vi "GeoData.vi"() -> ()   [LabVIEW 2017] (continued)
MI\tOttawa County\tH1\n49430\t26139\tLamont\tMI\tOttawa County\tH1\n49424\t26139\tHolland\tMI\tOttawa County\tH1\n49415\t26139\tFruitport\tMI\tOttawa County\tH1\n49434\t26139\tMacatawa\tMI\tOttawa County\tH1\n49315\t26139\tByron center\tMI\tOttawa County\tH1\n49330\t26139\tKent city\tMI\tOttawa County\tH1\n49534\t26139\tGrand rapids\tMI\tOttawa County\tH1\n49544\t26139\tGrand rapids\tMI\tOttawa County\tH1\n49422\t26139\tHolland\tMI\tOttawa County\tH1\n49464\t26139\tZeeland\tMI\tOttawa County\tH1\n49448\t26139\tNunica\tMI\tOttawa County\tH1\n49345\t26139\tSparta\tMI\tOttawa County\tH1\n49428\t26139\tJenison\tMI\tOttawa County\tH1\n49401\t26139\tAllendale\tMI\tOttawa County\tH1\n49435\t26139\tMarne\tMI\tOttawa County\tH1\n49404\t26139\tCoopersville\tMI\tOttawa County\tH1\n49417\t26139\tGrand haven\tMI\tOttawa County\tH1\n49460\t26139\tWest olive\tMI\tOttawa County\tH1\n49429\t26139\tJenison\tMI\tOttawa County\tH1\n49403\t26139\tConklin\tMI\tOttawa County\tH1\n49427\t26139\tJamestown\tMI\tOttawa County\tH1\n49318\t26139\tCasnovia\tMI\tOttawa County\tH1\n49451\t26139\tRavenna\tMI\tOttawa County\tH1\n49759\t26141\tMillersburg\tMI\tPresque Isle County\tH1\n49777\t26141\tPresque isle\tMI\tPresque Isle County\tH1\n49743\t26141\tHawks\tMI\tPresque Isle County\tH1\n49707\t26141\tAlpena\tMI\tPresque Isle County\tH1\n49721\t26141\tCheboygan\tMI\tPresque Isle County\tH1\n49746\t26141\tHillman\tMI\tPresque Isle County\tH1\n49776\t26141\tPosen\tMI\tPresque Isle County\tH1\n49779\t26141\tRogers city\tMI\tPresque Isle County\tH1\n49765\t26141\tOnaway\tMI\tPresque Isle County\tH1\n48629\t26143\tHoughton lake\tMI\tRoscommon County\tH1\n48624\t26143\tGladwin\tMI\tRoscommon County\tH1\n48627\t26143\tHiggins lake\tMI\tRoscommon County\tH1\n48653\t26143\tRoscommon\tMI\tRoscommon County\tH1\n48651\t26143\tPrudenville\tMI\tRoscommon County\tH1\n48630\t26143\tHoughton lake heights\tMI\tRoscommon County\tH1\n48656\t26143\tSaint helen\tMI\tRoscommon County\tH1\n48420\t26145\tClio\tMI\tSaginaw County\tH1\n48757\t26145\tReese\tMI\tSaginaw County\tH1\n48417\t26145\tBurt\tMI\tSaginaw County\tH1\n48623\t26145\tFreeland\tMI\tSaginaw County\tH1\n48734\t26145\tFrankenmuth\tMI\tSaginaw County\tH1\n48724\t26145\tCarrollton\tMI\tSaginaw County\tH1\n48457\t26145\tMontrose\tMI\tSaginaw County\tH1\n48601\t26145\tSaginaw\tMI\tSaginaw County\tH1\n48603\t26145\tSaginaw\tMI\tSaginaw County\tH1\n48708\t26145\tBay city\tMI\tSaginaw County\tH1\n48867\t26145\tOwosso\tMI\tSaginaw County\tH1\n48606\t26145\tSaginaw\tMI\tSaginaw County\tH1\n48787\t26145\tFrankenmuth\tMI\tSaginaw County\tH1\n48604\t26145\tSaginaw\tMI\tSaginaw County\tH1\n48608\t26145\tSaginaw\tMI\tSaginaw County\tH1\n48626\t26145\tHemlock\tMI\tSaginaw County\tH1\n48637\t26145\tMerrill\tMI\tSaginaw County\tH1\n48609\t26145\tSaginaw\tMI\tSaginaw County\tH1\n48747\t26145\tMunger\tMI\tSaginaw County\tH1\n48415\t26145\tBirch run\tMI\tSaginaw County\tH1\n48602\t26145\tSaginaw\tMI\tSaginaw County\tH1\n48638\t26145\tSaginaw\tMI\tSaginaw County\tH1\n48722\t26145\tBridgeport\tMI\tSaginaw County\tH1\n48649\t26145\tOakley\tMI\tSaginaw County\tH1\n48460\t26145\tNew lothrop\tMI\tSaginaw County\tH1\n48655\t26145\tSaint charles\tMI\tSaginaw County\tH1\n48607\t26145\tSaginaw\tMI\tSaginaw County\tH1\n48768\t26145\tVassar\tMI\tSaginaw County\tH1\n48841\t26145\tHenderson\tMI\tSaginaw County\tH1\n48616\t26145\tChesaning\tMI\tSaginaw County\tH1\n48807\t26145\tBannister\tMI\tSaginaw County\tH1\n48605\t26145\tSaginaw\tMI\tSaginaw County\tH1\n48614\t26145\tBrant\tMI\tSaginaw County\tH1\n48831\t26145\tElsie\tMI\tSaginaw County\tH1\n48663\t26145\tSaginaw\tMI\tSaginaw County\tH1\n48022\t26147\tEmmett\tMI\tSt. Clair County\tH1\n48014\t26147\tCapac\tMI\tSt. Clair County\tH1\n48041\t26147\tMemphis\tMI\tSt. Clair County\tH1\n48054\t26147\tEast china\tMI\tSt. Clair County\tH1\n48002\t26147\tAllenton\tMI\tSt. Clair County\tH1\n48064\t26147\tCasco\tMI\tSt. Clair County\tH1\n48049\t26147\tNorth street\tMI\tSt. Clair County\tH1\n48060\t26147\tPort huron\tMI\tSt. Clair County\tH1\n48444\t26147\tImlay city\tMI\tSt. Clair County\tH1\n48023\t26147\tFair haven\tMI\tSt. Clair County\tH1\n48032\t26147\tJeddo\tMI\tSt. Clair County\tH1\n48003\t26147\tAlmont\tMI\tSt. Clair County\tH1\n48027\t26147\tGoodells\tMI\tSt. Clair County\tH1\n48061\t26147\tPort huron\tMI\tSt. Clair County\tH1\n48040\t26147\tMarysville\tMI\tSt. Clair County\tH1\n48416\t26147\tBrown city\tMI\tSt. Clair County\tH1\n48006\t26147\tAvoca\tMI\tSt. Clair County\tH1\n48039\t26147\tMarine city\tMI\tSt. Clair County\tH1\n48001\t26147\tAlgonac\tMI\tSt. Clair County\tH1\n48028\t26147\tHarsens island\tMI\tSt. Clair County\tH1\n48004\t26147\tAnchorville\tMI\tSt. Clair County\tH1\n48097\t26147\tYale\tMI\tSt. Clair County\tH1\n48079\t26147\tSaint clair\tMI\tSt. Clair County\tH1\n48059\t26147\tFort gratiot\tMI\tSt. Clair County\tH1\n48074\t26147\tSmiths creek\tMI\tSt. Clair County\tH1\n48063\t26147\tColumbus\tMI\tSt. Clair County\tH1\n49040\t26149\tColon\tMI\tSt. Joseph County\tH1\n49099\t26149\tWhite pigeon\tMI\tSt. Joseph County\tH1\n49087\t26149\tSchoolcraft\tMI\tSt. Joseph County\tH1\n49042\t26149\tConstantine\tMI\tSt. Joseph County\tH1\n49011\t26149\tAthens\tMI\tSt. Joseph County\tH1\n49072\t26149\tMendon\tMI\tSt. Joseph County\tH1\n49075\t26149\tNottawa\tMI\tSt. Joseph County\tH1\n49093\t26149\tThree rivers\tMI\tSt. Joseph County\tH1\n49097\t26149\tVicksburg\tMI\tSt. Joseph County\tH1\n49091\t26149\tSturgis\tMI\tSt. Joseph County\tH1\n49052\t26149\tFulton\tMI\tSt. Joseph County\tH1\n49032\t26149\tCentreville\tMI\tSt. Joseph County\tH1\n49067\t26149\tMarcellus\tMI\tSt. Joseph County\tH1\n49030\t26149\tBurr oak\tMI\tSt. Joseph County\tH1\n49066\t26149\tLeonidas\tMI\tSt. Joseph County\tH1\n48427\t26151\tDeckerville\tMI\tSanilac County\tH1\n48456\t26151\tMinden city\tMI\tSanilac County\tH1\n48426\t26151\tDecker\tMI\tSanilac County\tH1\n48434\t26151\tForestville\tMI\tSanilac County\tH1\n48419\t26151\tCarsonville\tMI\tSanilac County\tH1\n48726\t26151\tCass city\tMI\tSanilac County\tH1\n48741\t26151\tKingston\tMI\tSanilac County\tH1\n48032\t26151\tJeddo\tMI\tSanilac County\tH1\n48422\t26151\tCroswell\tMI\tSanilac County\tH1\n48465\t26151\tPalms\tMI\tSanilac County\tH1\n48472\t26151\tSnover\tMI\tSanilac County\tH1\n48729\t26151\tDeford\tMI\tSanilac County\tH1\n48416\t26151\tBrown city\tMI\tSanilac County\tH1\n48453\t26151\tMarlette\tMI\tSanilac County\tH1\n48471\t26151\tSandusky\tMI\tSanilac County\tH1\n48450\t26151\tLexington\tMI\tSanilac County\tH1\n48401\t26151\tApplegate\tMI\tSanilac County\tH1\n48466\t26151\tPeck\tMI\tSanilac County\tH1\n48470\t26151\tRuth\tMI\tSanilac County\tH1\n48469\t26151\tPort sanilac\tMI\tSanilac County\tH1\n48097\t26151\tYale\tMI\tSanilac County\tH1\n48441\t26151\tHarbor beach\tMI\tSanilac County\tH1\n48475\t26151\tUbly\tMI\tSanilac County\tH1\n48454\t26151\tMelvin\tMI\tSanilac County\tH1\n48410\t26151\tArgyle\tMI\tSanilac County\tH1\n49817\t26153\tCooks\tMI\tSchoolcraft County\tH1\n49836\t26153\tGermfask\tMI\tSchoolcraft County\tH1\n49895\t26153\tWetmore\tMI\tSchoolcraft County\tH1\n49883\t26153\tSeney\tMI\tSchoolcraft County\tH1\n49884\t26153\tShingleton\tMI\tSchoolcraft County\tH1\n49854\t26153\tManistique\tMI\tSchoolcraft County\tH1\n49840\t26153\tGulliver\tMI\tSchoolcraft County\tH1\n48476\t26155\tVernon\tMI\tShiawassee County\tH1\n48414\t26155\tBancroft\tMI\tShiawassee County\tH1\n48840\t26155\tHaslett\tMI\tShiawassee County\tH1\n48429\t26155\tDurand\tMI\tShiawassee County\tH1\n48882\t26155\tShaftsburg\tMI\tShiawassee County\tH1\n48867\t26155\tOwosso\tMI\tShiawassee County\tH1\n48418\t26155\tByron\tMI\tShiawassee County\tH1\n48848\t26155\tLaingsburg\tMI\tShiawassee County\tH1\n48857\t26155\tMorrice\tMI\tShiawassee County\tH1\n48649\t26155\tOakley\tMI\tShiawassee County\tH1\n48836\t26155\tFowlerville\tMI\tShiawassee County\tH1\n48872\t26155\tPerry\tMI\tShiawassee County\tH1\n48460\t26155\tNew lothrop\tMI\tShiawassee County\tH1\n48433\t26155\tFlushing\tMI\tShiawassee County\tH1\n48436\t26155\tGaines\tMI\tShiawassee County\tH1\n48449\t26155\tLennon\tMI\tShiawassee County\tH1\n48817\t26155\tCorunna\tMI\tShiawassee County\tH1\n48841\t26155\tHenderson\tMI\tShiawassee County\tH1\n48616\t26155\tChesaning\tMI\tShiawassee County\tH1\n48866\t26155\tOvid\tMI\tShiawassee County\tH1\n48807\t26155\tBannister\tMI\tShiawassee County\tH1\n48831\t26155\tElsie\tMI\tShiawassee County\tH1\n48420\t26157\tClio\tMI\tTuscola County\tH1\n48757\t26157\tReese\tMI\tTuscola County\tH1\n48426\t26157\tDecker\tMI\tTuscola County\tH1\n48758\t26157\tRichville\tMI\tTuscola County\tH1\n48727\t26157\tClifford\tMI\tTuscola County\tH1\n48723\t26157\tCaro\tMI\tTuscola County\tH1\n48726\t26157\tCass city\tMI\tTuscola County\tH1\n48734\t26157\tFrankenmuth\tMI\tTuscola County\tH1\n48701\t26157\tAkron\tMI\tTuscola County\tH1\n48741\t26157\tKingston\tMI\tTuscola County\tH1\n48746\t26157\tMillington\tMI\tTuscola County\tH1\n48760\t26157\tSilverwood\tMI\tTuscola County\tH1\n48733\t26157\tFairgrove\tMI\tTuscola County\tH1\n48729\t26157\tDeford\tMI\tTuscola County\tH1\n48453\t26157\tMarlette\tMI\tTuscola County\tH1\n48735\t26157\tGagetown\tMI\tTuscola County\tH1\n48435\t26157\tFostoria\tMI\tTuscola County\tH1\n48744\t26157\tMayville\tMI\tTuscola County\tH1\n48759\t26157\tSebewaing\tMI\tTuscola County\tH1\n48464\t26157\tOtter lake\tMI\tTuscola County\tH1\n48415\t26157\tBirch run\tMI\tTuscola County\tH1\n48768\t26157\tVassar\tMI\tTuscola County\tH1\n48767\t26157\tUnionville\tMI\tTuscola County\tH1\n49043\t26159\tCovert\tMI\tVan Buren County\tH1\n49009\t26159\tKalamazoo\tMI\tVan Buren County\tH1\n49026\t26159\tBloomingdale\tMI\tVan Buren County\tH1\n49047\t26159\tDowagiac\tMI\tVan Buren County\tH1\n49090\t26159\tSouth haven\tMI\tVan Buren County\tH1\n49056\t26159\tGrand junction\tMI\tVan Buren County\tH1\n49087\t26159\tSchoolcraft\tMI\tVan Buren County\tH1\n49079\t26159\tPaw paw\tMI\tVan Buren County\tH1\n49098\t26159\tWatervliet\tMI\tVan Buren County\tH1\n49022\t26159\tBenton harbor\tMI\tVan Buren County\tH1\n49045\t26159\tDecatur\tMI\tVan Buren County\tH1\n49057\t26159\tHartford\tMI\tVan Buren County\tH1\n49063\t26159\tLacota\tMI\tVan Buren County\tH1\n49065\t26159\tLawton\tMI\tVan Buren County\tH1\n49078\t26159\tOtsego\tMI\tVan Buren County\tH1\n49062\t26159\tKendall\tMI\tVan Buren County\tH1\n49010\t26159\tAllegan\tMI\tVan Buren County\tH1\n49038\t26159\tColoma\tMI\tVan Buren County\tH1\n49067\t26159\tMarcellus\tMI\tVan Buren County\tH1\n49027\t26159\tBreedsville\tMI\tVan Buren County\tH1\n49013\t26159\tBangor\tMI\tVan Buren County\tH1\n49055\t26159\tGobles\tMI\tVan Buren County\tH1\n49071\t26159\tMattawan\tMI\tVan Buren County\tH1\n49064\t26159\tLawrence\tMI\tVan Buren County\tH1\n48137\t26161\tGregory\tMI\tWashtenaw County\tH1\n48178\t26161\tSouth lyon\tMI\tWashtenaw County\tH1\n49285\t26161\tStockbridge\tMI\tWashtenaw County\tH1\n48113\t26161\tAnn arbor\tMI\tWashtenaw County\tH1\n48175\t26161\tSalem\tMI\tWashtenaw County\tH1\n48111\t26161\tBelleville\tMI\tWashtenaw County\tH1\n48109\t26161\tAnn arbor\tMI\tWashtenaw County\tH1\n48107\t26161\tAnn arbor\tMI\tWashtenaw County\tH1\n48103\t26161\tAnn arbor\tMI\tWashtenaw County\tH1\n48130\t26161\tDexter\tMI\tWashtenaw County\tH1\n48169\t26161\tPinckney\tMI\tWashtenaw County\tH1\n48189\t26161\tWhitmore lake\tMI\tWashtenaw County\tH1\n48105\t26161\tAnn arbor\tMI\tWashtenaw County\tH1\n48108\t26161\tAnn arbor\tMI\tWashtenaw County\tH1\n48170\t26161\tPlymouth\tMI\tWashtenaw County\tH1\n48167\t26161\tNorthville\tMI\tWashtenaw County\tH1\n48168\t26161\tNorthville\tMI\tWashtenaw County\tH1\n49229\t26161\tBritton\tMI\tWashtenaw County\tH1\n49287\t26161\tTipton\tMI\tWashtenaw County\tH1\n48158\t26161\tManchester\tMI\tWashtenaw County\tH1\n48191\t26161\tWillis\tMI\tWashtenaw County\tH1\n48190\t26161\tWhittaker\tMI\tWashtenaw County\tH1\n48118\t26161\tChelsea\tMI\tWashtenaw County\tH1\n48160\t26161\tMilan\tMI\tWashtenaw County\tH1\n48104\t26161\tAnn arbor\tMI\tWashtenaw County\tH1\n48106\t26161\tAnn arbor\tMI\tWashtenaw County\tH1\n48197\t26161\tYpsilanti\tMI\tWashtenaw County\tH1\n48176\t26161\tSaline\tMI\tWashtenaw County\tH1\n49236\t26161\tClinton\tMI\tWashtenaw County\tH1\n48198\t26161\tYpsilanti\tMI\tWashtenaw County\tH1\n49230\t26161\tBrooklyn\tMI\tWashtenaw County\tH1\n49240\t26161\tGrass lake\tMI\tWashtenaw County\tH1\n48124\t26163\tDearborn\tMI\tWayne County\tH1\n48195\t26163\tSouthgate\tMI\tWayne County\tH1\n48201\t26163\tDetroit\tMI\tWayne County\tH1\n48212\t26163\tHamtramck\tMI\tWayne County\tH1\n48209\t26163\tDetroit\tMI\tWayne County\tH1\n48210\t26163\tDetroit\tMI\tWayne County\tH1\n48211\t26163\tDetroit\tMI\tWayne County\tH1\n48225\t26163\tHarper woods\tMI\tWayne County\tH1\n48226\t26163\tDetroit\tMI\tWayne County\tH1\n48080\t26163\tSaint clair shores\tMI\tWayne County\tH1\n48111\t26163\tBelleville\tMI\tWayne County\tH1\n48134\t26163\tFlat rock\tMI\tWayne County\tH1\n48152\t26163\tLivonia\tMI\tWayne County\tH1\n48193\t26163\tRiverview\tMI\tWayne County\tH1\n48235\t26163\tDetroit\tMI\tWayne County\tH1\n48221\t26163\tDetroit\tMI\tWayne County\tH1\n48230\t26163\tGrosse pointe\tMI\tWayne County\tH1\n48128\t26163\tDearborn\tMI\tWayne County\tH1\n48150\t26163\tLivonia\tMI\tWayne County\tH1\n48146\t26163\tLincoln park\tMI\tWayne County\tH1\n48164\t26163\tNew boston\tMI\tWayne County\tH1\n48125\t26163\tDearborn heights\tMI\tWayne County\tH1\n48186\t26163\tWestland\tMI\tWayne County\tH1\n48187\t26163\tCanton\tMI\tWayne County\tH1\n48185\t26163\tWestland\tMI\tWayne County\tH1\n48180\t26163\tTaylor\tMI\tWayne County\tH1\n48205\t26163\tDetroit\tMI\tWayne County\tH1\n48236\t26163\tGrosse pointe\tMI\tWayne County\tH1\n48214\t26163\tDetroit\tMI\tWayne County\tH1\n48242\t26163\tDetroit\tMI\tWayne County\tH1\n48151\t26163\tLivonia\tMI\tWayne County\tH1\n48136\t26163\tGarden city\tMI\tWayne County\tH1\n48222\t26163\tDetroit\tMI\tWayne County\tH1\n48126\t26163\tDearborn\tMI\tWayne County\tH1\n48127\t26163\tDearborn heights\tMI\tWayne County\tH1\n48170\t26163\tPlymouth\tMI\tWayne County\tH1\n48167\t26163\tNorthville\tMI\tWayne County\tH1\n48168\t26163\tNorthville\tMI\tWayne County\tH1\n48117\t26163\tCarleton\tMI\tWayne County\tH1\n48183\t26163\tTrenton\tMI\tWayne County\tH1\n48174\t26163\tRomulus\tMI\tWayne County\tH1\n48208\t26163\tDetroit\tMI\tWayne County\tH1\n48173\t26163\tRockwood\tMI\tWayne County\tH1\n48184\t26163\tWayne\tMI\tWayne County\tH1\n48204\t26163\tDetroit\tMI\tWayne County\tH1\n48244\t26163\tDetroit\tMI\tWayne County\tH1\n48120\t26163\tDearborn\tMI\tWayne County\tH1\n48188\t26163\tCanton\tMI\tWayne County\tH1\n48203\t26163\tHighland park\tMI\tWayne County\tH1\n48213\t26163\tDetroit\tMI\tWayne County\tH1\n48239\t26163\tRedford\tMI\tWayne County\tH1\n48234\t26163\tDetroit\tMI\tWayne County\tH1\n48238\t26163\tDetroit\tMI\tWayne County\tH1\n48233\t26163\tDetroit\tMI\tWayne County\tH1\n48138\t26163\tGrosse ile\tMI\tWayne County\tH1\n48101\t26163\tAllen park\tMI\tWayne County\tH1\n48135\t26163\tGarden city\tMI\tWayne County\tH1\n48202\t26163\tDetroit\tMI\tWayne County\tH1\n48207\t26163\tDetroit\tMI\tWayne County\tH1\n48075\t26163\tSouthfield\tMI\tWayne County\tH1\n48243\t26163\tDetroit\tMI\tWayne County\tH1\n48122\t26163\tMelvindale\tMI\tWayne County\tH1\n48141\t26163\tInkster\tMI\tWayne County\tH1\n48123\t26163\tDearborn\tMI\tWayne County\tH1\n48154\t26163\tLivonia\tMI\tWayne County\tH1\n48192\t26163\tWyandotte\tMI\tWayne County\tH1\n48206\t26163\tDetroit\tMI\tWayne County\tH1\n48216\t26163\tDetroit\tMI\tWayne County\tH1\n48228\t26163\tDetroit\tMI\tWayne County\tH1\n48219\t26163\tDetroit\tMI\tWayne County\tH1\n48229\t26163\tEcorse\tMI\tWayne County\tH1\n48231\t26163\tDetroit\tMI\tWayne County\tH1\n48153\t26163\tLivonia\tMI\tWayne County\tH1\n48227\t26163\tDetroit\tMI\tWayne County\tH1\n48240\t26163\tRedford\tMI\tWayne County\tH1\n48223\t26163\tDetroit\tMI\tWayne County\tH1\n48224\t26163\tDetroit\tMI\tWayne County\tH1\n48215\t26163\tDetroit\tMI\tWayne County\tH1\n48218\t26163\tRiver rouge\tMI\tWayne County\tH1\n48217\t26163\tDetroit\tMI\tWayne County\tH1\n48232\t26163\tDetroit\tMI\tWayne County\tH1\n48121\t26163\tDearborn\tMI\tWayne County\tH1\n48288\t26163\tDetroit\tMI\tWayne County\tH1\n49618\t26165\tBoon\tMI\tWexford County\tH1\n49638\t26165\tHarrietta\tMI\tWexford County\tH1\n49620\t26165\tBuckley\tMI\tWexford County\tH1\n49633\t26165\tFife lake\tMI\tWexford County\tH1\n49688\t26165\tTustin\tMI\tWexford County\tH1\n49601\t26165\tCadillac\tMI\tWexford County\tH1\n49689\t26165\tWellston\tMI\tWexford County\tH1\n49663\t26165\tManton\tMI\tWexford County\tH1\n49668\t26165\tMesick\tMI\tWexford County\tH1\n49625\t26165\tCopemish\tMI\tWexford County\tH1\n49649\t26165\tKingsley\tMI\tWexford County\tH1\n49657\t26165\tMc bain\tMI\tWexford County\tH1\n55798\t27001\tWright\tMN\tAitkin County\tH1\n55735\t27001\tFinlayson\tMN\tAitkin County\tH1\n56469\t27001\tPalisade\tMN\tAitkin County\tH1\n55787\t27001\tTamarack\tMN\tAitkin County\tH1\n56342\t27001\tIsle\tMN\tAitkin County\tH1\n56431\t27001\tAitkin\tMN\tAitkin County\tH1\n56350\t27001\tMc grath\tMN\tAitkin County\tH1\n55785\t27001\tSwatara\tMN\tAitkin County\tH1\n55760\t27001\tMcgregor\tMN\tAitkin County\tH1\n56444\t27001\tDeerwood\tMN\tAitkin County\tH1\n55752\t27001\tJacobson\tMN\tAitkin County\tH1\n55072\t27001\tSandstone\tMN\tAitkin County\tH1\n55748\t27001\tHill city\tMN\tAitkin County\tH1\n55783\t27001\tSturgeon lake\tMN\tAitkin County\tH1\n55014\t27003\tCircle pines\tMN\tAnoka County\tH1\n55126\t27003\tSaint paul\tMN\tAnoka County\tH1\n55303\t27003\tAnoka\tMN\tAnoka County\tH1\n55448\t27003\tMinneapolis\tMN\tAnoka County\tH1\n55092\t27003\tWyoming\tMN\tAnoka County\tH1\n55112\t27003\tSaint paul\tMN\tAnoka County\tH1\n55330\t27003\tElk river\tMN\tAnoka County\tH1\n55433\t27003\tMinneapolis\tMN\tAnoka County\tH1\n55025\t27003\tForest lake\tMN\tAnoka County\tH1\n55434\t27003\tMinneapolis\tMN\tAnoka County\tH1\n55449\t27003\tMinneapolis\tMN\tAnoka County\tH1\n55070\t27003\tSaint francis\tMN\tAnoka County\tH1\n55304\t27003\tAndover\tMN\tAnoka County\tH1\n55432\t27003\tMinneapolis\tMN\tAnoka County\tH1\n55398\t27003\tZimmerman\tMN\tAnoka County\tH1\n55421\t27003\tMinneapolis\tMN\tAnoka County\tH1\n55005\t27003\tBethel\tMN\tAnoka County\tH1\n55011\t27003\tCedar\tMN\tAnoka County\tH1\n55038\t27003\tHugo\tMN\tAnoka County\tH1\n55040\t27003\tIsanti\tMN\tAnoka County\tH1\n55079\t27003\tStacy\tMN\tAnoka County\tH1\n55110\t27003\tSaint paul\tMN\tAnoka County\tH1\n56570\t27005\tOsage\tMN\tBecker County\tH1\n56577\t27005\tRichwood\tMN\tBecker County\tH1\n56464\t27005\tMenahga\tMN\tBecker County\tH1\n56511\t27005\tAudubon\tMN\tBecker County\tH1\n56578\t27005\tRochert\tMN\tBecker County\tH1\n56585\t27005\tUlen\tMN\tBecker County\tH1\n56470\t27005\tPark rapids\tMN\tBecker County\tH1\n56477\t27005\tSebeka\tMN\tBecker County\tH1\n56549\t27005\tHawley\tMN\tBecker County\tH1\n56591\t27005\tWhite earth\tMN\tBecker County\tH1\n56589\t27005\tWaubun\tMN\tBecker County\tH1\n56554\t27005\tLake park\tMN\tBecker County\tH1\n56502\t27005\tDetroit lakes\tMN\tBecker County\tH1\n56552\t27005\tHitterdal\tMN\tBecker County\tH1\n56572\t27005\tPelican rapids\tMN\tBecker County\tH1\n56593\t27005\tWolf lake\tMN\tBecker County\tH1\n56501\t27005\tDetroit lakes\tMN\tBecker County\tH1\n56544\t27005\tFrazee\tMN\tBecker County\tH1\n56521\t27005\tCallaway\tMN\tBecker County\tH1\n56575\t27005\tPonsford\tMN\tBecker County\tH1\n56569\t27005\tOgema\tMN\tBecker County\tH1\n56678\t27007\tSolway\tMN\tBeltrami County\tH1\n56727\t27007\tGrygla\tMN\tBeltrami County\tH1\n56630\t27007\tBlackduck\tMN\tBeltrami County\tH1\n56633\t27007\tCass lake\tMN\tBeltrami County\tH1\n56619\t27007\tBemidji\tMN\tBeltrami County\tH1\n56666\t27007\tPonemah\tMN\tBeltrami County\tH1\n56661\t27007\tNorthome\tMN\tBeltrami County\tH1\n56670\t27007\tRedby\tMN\tBeltrami County\tH1\n56671\t27007\tRedlake\tMN\tBeltrami County\tH1\n56685\t27007\tWaskish\tMN\tBeltrami County\tH1\n56647\t27007\tHines\tMN\tBeltrami County\tH1\n56676\t27007\tShevlin\tMN\tBeltrami County\tH1\n56683\t27007\tTenstrike\tMN\tBeltrami County\tH1\n56601\t27007\tBemidji\tMN\tBeltrami County\tH1\n56650\t27007\tKelliher\tMN\tBeltrami County\tH1\n56663\t27007\tPennington\tMN\tBeltrami County\tH1\n56667\t27007\tPuposky\tMN\tBeltrami County\tH1\n56652\t27007\tLeonard\tMN\tBeltrami County\tH1\n56379\t27009\tSauk rapids\tMN\tBenton County\tH1\n56330\t27009\tForeston\tMN\tBenton County\tH1\n56303\t27009\tSaint cloud\tMN\tBenton County\tH1\n56377\t27009\tSartell\tMN\tBenton County\tH1\n56367\t27009\tRice\tMN\tBenton County\tH1\n56304\t27009\tSaint cloud\tMN\tBenton County\tH1\n56387\t27009\tWaite park\tMN\tBenton County\tH1\n55371\t27009\tPrinceton\tMN\tBenton County\tH1\n56373\t27009\tRoyalton\tMN\tBenton County\tH1\n56357\t27009\tOak park\tMN\tBenton County\tH1\n56333\t27009\tGilman\tMN\tBenton County\tH1\n56329\t27009\tFoley\tMN\tBenton County\tH1\n56219\t27011\tBrowns valley\tMN\tBig Stone County\tH1\n56236\t27011\tDumont\tMN\tBig Stone County\tH1\n56225\t27011\tClinton\tMN\tBig Stone County\tH1\n56227\t27011\tCorrell\tMN\tBig Stone County\tH1\n56278\t27011\tOrtonville\tMN\tBig Stone County\tH1\n56211\t27011\tBeardsley\tMN\tBig Stone County\tH1\n56208\t27011\tAppleton\tMN\tBig Stone County\tH1\n56240\t27011\tGraceville\tMN\tBig Stone County\tH1\n56210\t27011\tBarry\tMN\tBig Stone County\tH1\n56221\t27011\tChokio\tMN\tBig Stone County\tH1\n56276\t27011\tOdessa\tMN\tBig Stone County\tH1\n56090\t27013\tVernon center\tMN\tBlue Earth County\tH1\n56080\t27013\tSaint clair\tMN\tBlue Earth County\tH1\n56024\t27013\tEagle lake\tMN\tBlue Earth County\tH1\n56034\t27013\tGarden city\tMN\tBlue Earth County\tH1\n56068\t27013\tMinnesota lake\tMN\tBlue Earth County\tH1\n56050\t27013\tKasota\tMN\tBlue Earth County\tH1\n56037\t27013\tGood thunder\tMN\tBlue Earth County\tH1\n56078\t27013\tPemberton\tMN\tBlue Earth County\tH1\n56063\t27013\tMadison lake\tMN\tBlue Earth County\tH1\n56001\t27013\tMankato\tMN\tBlue Earth County\tH1\n56062\t27013\tMadelia\tMN\tBlue Earth County\tH1\n56041\t27013\tHanska\tMN\tBlue Earth County\tH1\n56003\t27013\tMankato\tMN\tBlue Earth County\tH1\n56073\t27013\tNew ulm\tMN\tBlue Earth County\tH1\n56065\t27013\tMapleton\tMN\tBlue Earth County\tH1\n56025\t27013\tEaston\tMN\tBlue Earth County\tH1\n56010\t27013\tAmboy\tMN\tBlue Earth County\tH1\n56060\t27013\tLewisville\tMN\tBlue Earth County\tH1\n56055\t27013\tLake crystal\tMN\tBlue Earth County\tH1\n56088\t27013\tTruman\tMN\tBlue Earth County\tH1\n56048\t27013\tJanesville\tMN\tBlue Earth County\tH1\n55333\t27015\tFranklin\tMN\tBrown County\tH1\n56081\t27015\tSaint james\tMN\tBrown County\tH1\n56266\t27015\tMorgan\tMN\tBrown County\tH1\n56085\t27015\tSleepy eye\tMN\tBrown County\tH1\n56087\t27015\tSpringfield\tMN\tBrown County\tH1\n56062\t27015\tMadelia\tMN\tBrown County\tH1\n56041\t27015\tHanska\tMN\tBrown County\tH1\n56019\t27015\tComfrey\tMN\tBrown County\tH1\n56030\t27015\tEssig\tMN\tBrown County\tH1\n56084\t27015\tSearles\tMN\tBrown County\tH1\n56073\t27015\tNew ulm\tMN\tBrown County\tH1\n56083\t27015\tSanborn\tMN\tBrown County\tH1\n55798\t27017\tWright\tMN\tCarlton County\tH1\n55797\t27017\tWrenshall\tMN\tCarlton County\tH1\n55736\t27017\tFloodwood\tMN\tCarlton County\tH1\n55780\t27017\tSawyer\tMN\tCarlton County\tH1\n55720\t27017\tCloquet\tMN\tCarlton County\tH1\n55787\t27017\tTamarack\tMN\tCarlton County\tH1\n55749\t27017\tHolyoke\tMN\tCarlton County\tH1\n55756\t27017\tKerrick\tMN\tCarlton County\tH1\n55726\t27017\tCromwell\tMN\tCarlton County\tH1\n55718\t27017\tCarlton\tMN\tCarlton County\tH1\n55810\t27017\tDuluth\tMN\tCarlton County\tH1\n55733\t27017\tEsko\tMN\tCarlton County\tH1\n55767\t27017\tMoose lake\tMN\tCarlton County\tH1\n55757\t27017\tKettle river\tMN\tCarlton County\tH1\n55707\t27017\tBarnum\tMN\tCarlton County\tH1\n55783\t27017\tSturgeon lake\tMN\tCarlton County\tH1\n55331\t27019\tExcelsior\tMN\tCarver County\tH1\n55386\t27019\tVictoria\tMN\tCarver County\tH1\n55363\t27019\tMontrose\tMN\tCarver County\tH1\n55368\t27019\tNorwood young america\tMN\tCarver County\tH1\n55339\t27019\tHamburg\tMN\tCarver County\tH1\n55317\t27019\tChanhassen\tMN\tCarver County\tH1\n55338\t27019\tGreen isle\tMN\tCarver County\tH1\n55322\t27019\tCologne\tMN\tCarver County\tH1\n55328\t27019\tDelano\tMN\tCarver County\tH1\n55388\t27019\tWatertown\tMN\tCarver County\tH1\n55318\t27019\tChaska\tMN\tCarver County\tH1\n55387\t27019\tWaconia\tMN\tCarver County\tH1\n56011\t27019\tBelle plaine\tMN\tCarver County\tH1\n55375\t27019\tSaint bonifacius\tMN\tCarver County\tH1\n55367\t27019\tNew germany\tMN\tCarver County\tH1\n55397\t27019\tYoung america\tMN\tCarver County\tH1\n55395\t27019\tWinsted\tMN\tCarver County\tH1\n55315\t27019\tCarver\tMN\tCarver County\tH1\n55360\t27019\tMayer\tMN\tCarver County\tH1\n56636\t27021\tDeer river\tMN\tCass County\tH1\n56472\t27021\tPequot lakes\tMN\tCass County\tH1\n56481\t27021\tVerndale\tMN\tCass County\tH1\n56464\t27021\tMenahga\tMN\tCass County\tH1\n56461\t27021\tLaporte\tMN\tCass County\tH1\n56468\t27021\tNisswa\tMN\tCass County\tH1\n56633\t27021\tCass lake\tMN\tCass County\tH1\n56425\t27021\tBaxter\tMN\tCass County\tH1\n56479\t27021\tStaples\tMN\tCass County\tH1\n56452\t27021\tHackensack\tMN\tCass County\tH1\n56401\t27021\tBrainerd\tMN\tCass County\tH1\n56672\t27021\tRemer\tMN\tCass County\tH1\n56477\t27021\tSebeka\tMN\tCass County\tH1\n55785\t27021\tSwatara\tMN\tCass County\tH1\n56473\t27021\tPillager\tMN\tCass County\tH1\n56601\t27021\tBemidji\tMN\tCass County\tH1\n56466\t27021\tMotley\tMN\tCass County\tH1\n56662\t27021\tOuting\tMN\tCass County\tH1\n56641\t27021\tFederal dam\tMN\tCass County\tH1\n56655\t27021\tLongville\tMN\tCass County\tH1\n56626\t27021\tBena\tMN\tCass County\tH1\n56474\t27021\tPine river\tMN\tCass County\tH1\n56484\t27021\tWalker\tMN\tCass County\tH1\n56433\t27021\tAkeley\tMN\tCass County\tH1\n56435\t27021\tBackus\tMN\tCass County\tH1\n56448\t27021\tFifty lakes\tMN\tCass County\tH1\n56295\t27023\tWatson\tMN\tChippewa County\tH1\n56241\t27023\tGranite falls\tMN\tChippewa County\tH1\n56252\t27023\tKerkhoven\tMN\tChippewa County\tH1\n56265\t27023\tMontevideo\tMN\tChippewa County\tH1\n56208\t27023\tAppleton\tMN\tChippewa County\tH1\n56262\t27023\tMilan\tMN\tChippewa County\tH1\n56260\t27023\tMaynard\tMN\tChippewa County\tH1\n56285\t27023\tSacred heart\tMN\tChippewa County\tH1\n56271\t27023\tMurdock\tMN\tChippewa County\tH1\n56282\t27023\tRaymond\tMN\tChippewa County\tH1\n56215\t27023\tBenson\tMN\tChippewa County\tH1\n56222\t27023\tClara city\tMN\tChippewa County\tH1\n55069\t27025\tRush city\tMN\tChisago County\tH1\n55074\t27025\tShafer\tMN\tChisago County\tH1\n55092\t27025\tWyoming\tMN\tChisago County\tH1\n55045\t27025\tLindstrom\tMN\tChisago County\tH1\n55013\t27025\tChisago city\tMN\tChisago County\tH1\n55032\t27025\tHarris\tMN\tChisago County\tH1\n55080\t27025\tStanchfield\tMN\tChisago County\tH1\n55084\t27025\tTaylors falls\tMN\tChisago County\tH1\n55008\t27025\tCambridge\tMN\tChisago County\tH1\n55025\t27025\tForest lake\tMN\tChisago County\tH1\n55006\t27025\tBraham\tMN\tChisago County\tH1\n55056\t27025\tNorth branch\tMN\tChisago County\tH1\n55073\t27025\tScandia\tMN\tChisago County\tH1\n55012\t27025\tCenter city\tMN\tChisago County\tH1\n55079\t27025\tStacy\tMN\tChisago County\tH1\n56584\t27027\tTwin valley\tMN\tClay County\tH1\n56561\t27027\tMoorhead\tMN\tClay County\tH1\n56585\t27027\tUlen\tMN\tClay County\tH1\n56562\t27027\tMoorhead\tMN\tClay County\tH1\n56580\t27027\tSabin\tMN\tClay County\tH1\n56547\t27027\tGlyndon\tMN\tClay County\tH1\n56529\t27027\tDilworth\tMN\tClay County\tH1\n56594\t27027\tWolverton\tMN\tClay County\tH1\n56549\t27027\tHawley\tMN\tClay County\tH1\n56574\t27027\tPerley\tMN\tClay County\tH1\n56546\t27027\tGeorgetown\tMN\tClay County\tH1\n56554\t27027\tLake park\tMN\tClay County\tH1\n56519\t27027\tBorup\tMN\tClay County\tH1\n56552\t27027\tHitterdal\tMN\tClay County\tH1\n56514\t27027\tBarnesville\tMN\tClay County\tH1\n56572\t27027\tPelican rapids\tMN\tClay County\tH1\n56563\t27027\tMoorhead\tMN\tClay County\tH1\n56525\t27027\tComstock\tMN\tClay County\tH1\n56536\t27027\tFelton\tMN\tClay County\tH1\n56560\t27027\tMoorhead\tMN\tClay County\tH1\n56678\t27029\tSolway\tMN\tClearwater County\tH1\n56470\t27029\tPark rapids\tMN\tClearwater County\tH1\n56621\t27029\tBagley\tMN\tClearwater County\tH1\n56676\t27029\tShevlin\tMN\tClearwater County\tH1\n56646\t27029\tGully\tMN\tClearwater County\tH1\n56557\t27029\tMahnomen\tMN\tClearwater County\tH1\n56644\t27029\tGonvick\tMN\tClearwater County\tH1\n56634\t27029\tClearbrook\tMN\tClearwater County\tH1\n56652\t27029\tLeonard\tMN\tClearwater County\tH1\n55612\t27031\tLutsen\tMN\tCook County\tH1\n55604\t27031\tGrand marais\tMN\tCook County\tH1\n55606\t27031\tHovland\tMN\tCook County\tH1\n55605\t27031\tGrand portage\tMN\tCook County\tH1\n55613\t27031\tSchroeder\tMN\tCook County\tH1\n55615\t27031\tTofte\tMN\tCook County\tH1\n56180\t27033\tWalnut grove\tMN\tCottonwood County\tH1\n56166\t27033\tRevere\tMN\tCottonwood County\tH1\n56159\t27033\tMountain lake\tMN\tCottonwood County\tH1\n56137\t27033\tHeron lake\tMN\tCottonwood County\tH1\n56174\t27033\tStorden\tMN\tCottonwood County\tH1\n56152\t27033\tLamberton\tMN\tCottonwood County\tH1\n56087\t27033\tSpringfield\tMN\tCottonwood County\tH1\n56131\t27033\tFulda\tMN\tCottonwood County\tH1\n56019\t27033\tComfrey\tMN\tCottonwood County\tH1\n56145\t27033\tJeffers\tMN\tCottonwood County\tH1\n56083\t27033\tSanborn\tMN\tCottonwood County\tH1\n56101\t27033\tWindom\tMN\tCottonwood County\tH1\n56183\t27033\tWestbrook\tMN\tCottonwood County\tH1\n56118\t27033\tBingham lake\tMN\tCottonwood County\tH1\n56364\t27035\tPierz\tMN\tCrow Wing County\tH1\n56472\t27035\tPequot lakes\tMN\tCrow Wing County\tH1\n56468\t27035\tNisswa\tMN\tCrow Wing County\tH1\n56425\t27035\tBaxter\tMN\tCrow Wing County\tH1\n56431\t27035\tAitkin\tMN\tCrow Wing County\tH1\n56441\t27035\tCrosby\tMN\tCrow Wing County\tH1\n56338\t27035\tHillman\tMN\tCrow Wing County\tH1\n56401\t27035\tBrainerd\tMN\tCrow Wing County\tH1\n56447\t27035\tEmily\tMN\tCrow Wing County\tH1\n56442\t27035\tCrosslake\tMN\tCrow Wing County\tH1\n56444\t27035\tDeerwood\tMN\tCrow Wing County\tH1\n56449\t27035\tFort ripley\tMN\tCrow Wing County\tH1\n56450\t27035\tGarrison\tMN\tCrow Wing County\tH1\n56455\t27035\tIronton\tMN\tCrow Wing County\tH1\n56662\t27035\tOuting\tMN\tCrow Wing County\tH1\n56465\t27035\tMerrifield\tMN\tCrow Wing County\tH1\n56474\t27035\tPine river\tMN\tCrow Wing County\tH1\n56435\t27035\tBackus\tMN\tCrow Wing County\tH1\n56448\t27035\tFifty lakes\tMN\tCrow Wing County\tH1\n55306\t27037\tBurnsville\tMN\tDakota County\tH1\n55121\t27037\tSaint paul\tMN\tDakota County\tH1\n55337\t27037\tBurnsville\tMN\tDakota County\tH1\n55089\t27037\tWelch\tMN\tDakota County\tH1\n55010\t27037\tCastle rock\tMN\tDakota County\tH1\n55033\t27037\tHastings\tMN\tDakota County\tH1\n55057\t27037\tNorthfield\tMN\tDakota County\tH1\n55124\t27037\tSaint paul\tMN\tDakota County\tH1\n55118\t27037\tSaint paul\tMN\tDakota County\tH1\n55009\t27037\tCannon falls\tMN\tDakota County\tH1\n55076\t27037\tInver grove heights\tMN\tDakota County\tH1\n55077\t27037\tInver grove heights\tMN\tDakota County\tH1\n55109\t27037\tSaint paul\tMN\tDakota County\tH1\n55044\t27037\tLakeville\tMN\tDakota County\tH1\n55068\t27037\tRosemount\tMN\tDakota County\tH1\n55120\t27037\tSaint paul\tMN\tDakota County\tH1\n55123\t27037\tSaint paul\tMN\tDakota County\tH1\n55065\t27037\tRandolph\tMN\tDakota County\tH1\n55031\t27037\tHampton\tMN\tDakota County\tH1\n55122\t27037\tSaint paul\tMN\tDakota County\tH1\n55018\t27037\tDennison\tMN\tDakota County\tH1\n55024\t27037\tFarmington\tMN\tDakota County\tH1\n55075\t27037\tSouth saint paul\tMN\tDakota County\tH1\n55085\t27037\tVermillion\tMN\tDakota County\tH1\n55150\t27037\tMendota\tMN\tDakota County\tH1\n55944\t27039\tKasson\tMN\tDodge County\tH1\n55924\t27039\tClaremont\tMN\tDodge County\tH1\n55946\t27039\tKenyon\tMN\tDodge County\tH1\n55955\t27039\tMantorville\tMN\tDodge County\tH1\n55917\t27039\tBlooming prairie\tMN\tDodge County\tH1\n55920\t27039\tByron\tMN\tDodge County\tH1\n55985\t27039\tWest concord\tMN\tDodge County\tH1\n55973\t27039\tSargeant\tMN\tDodge County\tH1\n55927\t27039\tDodge center\tMN\tDodge County\tH1\n55940\t27039\tHayfield\tMN\tDodge County\tH1\n55963\t27039\tPine island\tMN\tDodge County\tH1\n55982\t27039\tWaltham\tMN\tDodge County\tH1\n56343\t27041\tKensington\tMN\tDouglas County\tH1\n56349\t27041\tLowry\tMN\tDouglas County\tH1\n56315\t27041\tBrandon\tMN\tDouglas County\tH1\n56334\t27041\tGlenwood\tMN\tDouglas County\tH1\n56308\t27041\tAlexandria\tMN\tDouglas County\tH1\n56319\t27041\tCarlos\tMN\tDouglas County\tH1\n56360\t27041\tOsakis\tMN\tDouglas County\tH1\n56309\t27041\tAshby\tMN\tDouglas County\tH1\n56361\t27041\tParkers prairie\tMN\tDouglas County\tH1\n56326\t27041\tEvansville\tMN\tDouglas County\tH1\n56332\t27041\tGarfield\tMN\tDouglas County\tH1\n56341\t27041\tHolmes city\tMN\tDouglas County\tH1\n56354\t27041\tMiltona\tMN\tDouglas County\tH1\n56446\t27041\tEagle bend\tMN\tDouglas County\tH1\n56327\t27041\tFarwell\tMN\tDouglas County\tH1\n56355\t27041\tNelson\tMN\tDouglas County\tH1\n56339\t27041\tHoffman\tMN\tDouglas County\tH1\n56385\t27041\tVillard\tMN\tDouglas County\tH1\n56098\t27043\tWinnebago\tMN\tFaribault County\tH1\n56027\t27043\tElmore\tMN\tFaribault County\tH1\n56047\t27043\tHuntley\tMN\tFaribault County\tH1\n56033\t27043\tFrost\tMN\tFaribault County\tH1\n56068\t27043\tMinnesota lake\tMN\tFaribault County\tH1\n56072\t27043\tNew richland\tMN\tFaribault County\tH1\n56051\t27043\tKiester\tMN\tFaribault County\tH1\n56009\t27043\tAlden\tMN\tFaribault County\tH1\n56023\t27043\tDelavan\tMN\tFaribault County\tH1\n56014\t27043\tBricelyn\tMN\tFaribault County\tH1\n56065\t27043\tMapleton\tMN\tFaribault County\tH1\n56013\t27043\tBlue earth\tMN\tFaribault County\tH1\n56025\t27043\tEaston\tMN\tFaribault County\tH1\n56039\t27043\tGranada\tMN\tFaribault County\tH1\n56010\t27043\tAmboy\tMN\tFaribault County\tH1\n56097\t27043\tWells\tMN\tFaribault County\tH1\n55975\t27045\tSpring valley\tMN\tFillmore County\tH1\n55923\t27045\tChatfield\tMN\tFillmore County\tH1\n55939\t27045\tHarmony\tMN\tFillmore County\tH1\n55951\t27045\tLe roy\tMN\tFillmore County\tH1\n55971\t27045\tRushford\tMN\tFillmore County\tH1\n55962\t27045\tPeterson\tMN\tFillmore County\tH1\n55967\t27045\tRacine\tMN\tFillmore County\tH1\n55979\t27045\tUtica\tMN\tFillmore County\tH1\n55990\t27045\tWykoff\tMN\tFillmore County\tH1\n55949\t27045\tLanesboro\tMN\tFillmore County\tH1\n55954\t27045\tMabel\tMN\tFillmore County\tH1\n55974\t27045\tSpring grove\tMN\tFillmore County\tH1\n55976\t27045\tStewartville\tMN\tFillmore County\tH1\n55961\t27045\tOstrander\tMN\tFillmore County\tH1\n55965\t27045\tPreston\tMN\tFillmore County\tH1\n55922\t27045\tCanton\tMN\tFillmore County\tH1\n55935\t27045\tFountain\tMN\tFillmore County\tH1\n56016\t27047\tClarks grove\tMN\tFreeborn County\tH1\n55917\t27047\tBlooming prairie\tMN\tFreeborn County\tH1\n56026\t27047\tEllendale\tMN\tFreeborn County\tH1\n56089\t27047\tTwin lakes\tMN\tFreeborn County\tH1\n56072\t27047\tNew richland\tMN\tFreeborn County\tH1\n56029\t27047\tEmmons\tMN\tFreeborn County\tH1\n56042\t27047\tHartland\tMN\tFreeborn County\tH1\n56043\t27047\tHayward\tMN\tFreeborn County\tH1\n56051\t27047\tKiester\tMN\tFreeborn County\tH1\n56009\t27047\tAlden\tMN\tFreeborn County\tH1\n56035\t27047\tGeneva\tMN\tFreeborn County\tH1\n56032\t27047\tFreeborn\tMN\tFreeborn County\tH1\n55912\t27047\tAustin\tMN\tFreeborn County\tH1\n56036\t27047\tGlenville\tMN\tFreeborn County\tH1\n56045\t27047\tHollandale\tMN\tFreeborn County\tH1\n56007\t27047\tAlbert lea\tMN\tFreeborn County\tH1\n56097\t27047\tWells\tMN\tFreeborn County\tH1\n55953\t27047\tLyle\tMN\tFreeborn County\tH1\n56020\t27047\tConger\tMN\tFreeborn County\tH1\n55992\t27049\tZumbrota\tMN\tGoodhue County\tH1\n55026\t27049\tFrontenac\tMN\tGoodhue County\tH1\n55089\t27049\tWelch\tMN\tGoodhue County\tH1\n55946\t27049\tKenyon\tMN\tGoodhue County\tH1\n55033\t27049\tHastings\tMN\tGoodhue County\tH1\n55041\t27049\tLake city\tMN\tGoodhue County\tH1\n55057\t27049\tNorthfield\tMN\tGoodhue County\tH1\n55985\t27049\tWest concord\tMN\tGoodhue County\tH1\n55027\t27049\tGoodhue\tMN\tGoodhue County\tH1\n55066\t27049\tRed wing\tMN\tGoodhue County\tH1\n55009\t27049\tCannon falls\tMN\tGoodhue County\tH1\n55956\t27049\tMazeppa\tMN\tGoodhue County\tH1\n55983\t27049\tWanamingo\tMN\tGoodhue County\tH1\n55963\t27049\tPine island\tMN\tGoodhue County\tH1\n55065\t27049\tRandolph\tMN\tGoodhue County\tH1\n55018\t27049\tDennison\tMN\tGoodhue County\tH1\n55053\t27049\tNerstrand\tMN\tGoodhue County\tH1\n56531\t27051\tElbow lake\tMN\tGrant County\tH1\n56274\t27051\tNorcross\tMN\tGrant County\tH1\n56248\t27051\tHerman\tMN\tGrant County\tH1\n56590\t27051\tWendell\tMN\tGrant County\tH1\n56309\t27051\tAshby\tMN\tGrant County\tH1\n56326\t27051\tEvansville\tMN\tGrant County\tH1\n56522\t27051\tCampbell\tMN\tGrant County\tH1\n56324\t27051\tDalton\tMN\tGrant County\tH1\n56235\t27051\tDonnelly\tMN\tGrant County\tH1\n56311\t27051\tBarrett\tMN\tGrant County\tH1\n56339\t27051\tHoffman\tMN\tGrant County\tH1\n56537\t27051\tFergus falls\tMN\tGrant County\tH1\n55107\t27053\tSaint paul\tMN\tHennepin County\tH1\n55113\t27053\tSaint paul\tMN\tHennepin County\tH1\n55331\t27053\tExcelsior\tMN\tHennepin County\tH1\n55343\t27053\tHopkins\tMN\tHennepin County\tH1\n55402\t27053\tMinneapolis\tMN\tHennepin County\tH1\n55435\t27053\tMinneapolis\tMN\tHennepin County\tH1\n55431\t27053\tMinneapolis\tMN\tHennepin County\tH1\n55439\t27053\tMinneapolis\tMN\tHennepin County\tH1\n55447\t27053\tMinneapolis\tMN\tHennepin County\tH1\n55386\t27053\tVictoria\tMN\tHennepin County\tH1\n55316\t27053\tChamplin\tMN\tHennepin County\tH1\n55341\t27053\tHanover\tMN\tHennepin County\tH1\n55327\t27053\tDayton\tMN\tHennepin County\tH1\n55364\t27053\tMound\tMN\tHennepin County\tH1\n55405\t27053\tMinneapolis\tMN\tHennepin County\tH1\n55406\t27053\tMinneapolis\tMN\tHennepin County\tH1\n55409\t27053\tMinneapolis\tMN\tHennepin County\tH1\n55359\t27053\tMaple plain\tMN\tHennepin County\tH1\n55426\t27053\tMinneapolis\tMN\tHennepin County\tH1\n55441\t27053\tMinneapolis\tMN\tHennepin County\tH1\n55446\t27053\tMinneapolis\tMN\tHennepin County\tH1\n55444\t27053\tMinneapolis\tMN\tHennepin County\tH1\n55417\t27053\tMinneapolis\tMN\tHennepin County\tH1\n55479\t27053\tMinneapolis\tMN\tHennepin County\tH1\n55330\t27053\tElk river\tMN\tHennepin County\tH1\n55428\t27053\tMinneapolis\tMN\tHennepin County\tH1\n55413\t27053\tMinneapolis\tMN\tHennepin County\tH1\n55418\t27053\tMinneapolis\tMN\tHennepin County\tH1\n55445\t27053\tMinneapolis\tMN\tHennepin County\tH1\n55111\t27053\tSaint paul\tMN\tHennepin County\tH1\n55361\t27053\tMinnetonka beach\tMN\tHennepin County\tH1\n55317\t27053\tChanhassen\tMN\tHennepin County\tH1\n55340\t27053\tHamel\tMN\tHennepin County\tH1\n55328\t27053\tDelano\tMN\tHennepin County\tH1\n55373\t27053\tRockford\tMN\tHennepin County\tH1\n55345\t27053\tMinnetonka\tMN\tHennepin County\tH1\n55388\t27053\tWatertown\tMN\tHennepin County\tH1\n55403\t27053\tMinneapolis\tMN\tHennepin County\tH1\n55408\t27053\tMinneapolis\tMN\tHennepin County\tH1\n55443\t27053\tMinneapolis\tMN\tHennepin County\tH1\n55440\t27053\tMinneapolis\tMN\tHennepin County\tH1\n55374\t27053\tRogers\tMN\tHennepin County\tH1\n55387\t27053\tWaconia\tMN\tHennepin County\tH1\n55346\t27053\tEden prairie\tMN\tHennepin County\tH1\n55437\t27053\tMinneapolis\tMN\tHennepin County\tH1\n55425\t27053\tMinneapolis\tMN\tHennepin County\tH1\n55458\t27053\tMinneapolis\tMN\tHennepin County\tH1\n55455\t27053\tMinneapolis\tMN\tHennepin County\tH1\n55487\t27053\tMinneapolis\tMN\tHennepin County\tH1\n55311\t27053\tMaple grove\tMN\tHennepin County\tH1\n55384\t27053\tSpring park\tMN\tHennepin County\tH1\n55401\t27053\tMinneapolis\tMN\tHennepin County\tH1\n55375\t27053\tSaint bonifacius\tMN\tHennepin County\tH1\n55410\t27053\tMinneapolis\tMN\tHennepin County\tH1\n55344\t27053\tEden prairie\tMN\tHennepin County\tH1\n55421\t27053\tMinneapolis\tMN\tHennepin County\tH1\n55438\t27053\tMinneapolis\tMN\tHennepin County
